vi "get_local_version.vi"(8 "error in (no error)":errorcluster, 11 "HelioUpdateMH100803 in":refnum<class "HelioUpdateMH100803.lvclass">) -> (0 "error out":errorcluster, 1 "file loading failed?":bool, 2 "local version out":string, 3 "HelioUpdateMH100803 out":refnum<class "HelioUpdateMH100803.lvclass">)   [LabVIEW 2010, in "HelioUpdateMH100803.lvclass"]
uses:
  HelioUpdateMH100803.lvclass
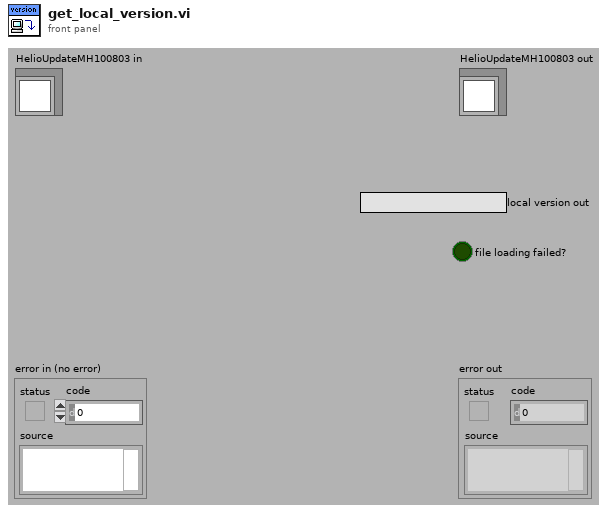
[diagram p1: front panel]
types:
  T1 = enum16{"open", "replace", "create", "open or create", "replace or create", "replace or create with confirmation"}
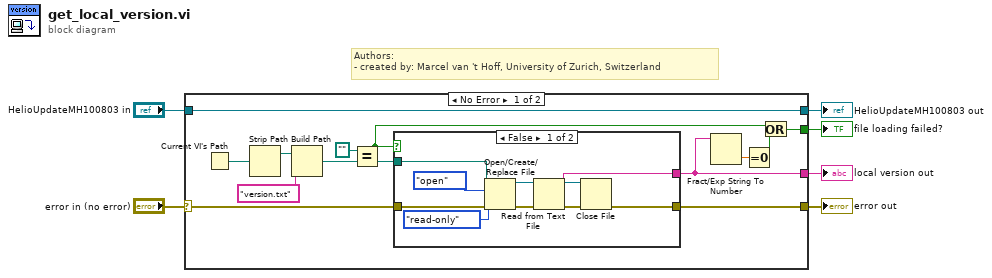
[diagram p0: block diagram]
diagram:
  # "Authors: \n- created by: Marcel van 't Hoff, University of Zurich, Switzerland"
  n1 = case shown="No Error" "error in (no error)" {
    selector: "error in (no error)" -> [w18 w32]
    tunnel: [w17 w32] -> w5
    tunnel: [w19 w31] -> w3
    tunnel: "HelioUpdateMH100803 in" -> [w19 w31]
    tunnel: [w7 _] -> w2
    tunnel: [w15 _] -> w1
    frame No Error {
      n2 = Current VI's Path() -> (path=w10:path)
      n3 = Strip Path(path=w10) -> (stripped path=w12:path)  [unwired: 1 out]
      n4 = Build Path(base path=w12, name or relative path="version.txt") -> (appended path=w9:path)
      n5 = Equal?(x=path "", y=w9) -> (x = y?=w14:bool)
      n6 = case shown="False" w14 {
        tunnel: w18 -> [w27 w30]
        tunnel: [w22 w30] -> w17
        tunnel: [w20 _] -> w7
        tunnel: w9 -> [w24 _]
        frame False {
          n7 = Open/Create/Replace File(file path (use dialog)=w24, error in=w27, operation (0:open)=T1."open", access (0:read/write)=enum16{"read/write", "read-only", "write-only"}."read-only") -> (refnum out=w29:refnum<file>, error out=w28:errorcluster)  [unwired: 2 in, 1 out]
          n8 = Read from Text File(file (use dialog)=w29, error in=w28) -> (refnum out=w21:refnum<file>, text=w20:string, error out=w23:errorcluster)  [unwired: 2 in, 1 out]
          n9 = Close File(refnum=w21, error in=w23) -> (error out=w22:errorcluster)  [unwired: 1 out]
        }
        frame True {
        }
      }
      n10 = Fract/Exp String To Number(string=w7) -> (number=w8:dbl)  [unwired: 3 in, 1 out]
      n11 = Equal To 0?(x=w8) -> (x = 0?=w13:bool)
      n12 = Or(x=w14, y=w13) -> (x .or. y?=w15:bool)
    }
    frame Error {
    }
  }
  "error out" <- w5
  "HelioUpdateMH100803 out" <- w3
  "local version out" <- w2
  "file loading failed?" <- w1
